vi "Ref_monitordata_struct_Add.vi"(6 "Active Sensors":bool[](array[boolean]), 8 "错误输入（无错误）":errorcluster, 9 "Controls[]":refnum<vi>[](array[refnum]), 10 "Ref_monitordata_struct":refnum<k24>[](array[refnum])) -> (0 "错误输出":errorcluster, 1 "Ref_monitordata_struct":refnum<k24>[](array[refnum]))   [LabVIEW 2017]
doc: "for reference monitor data"
uses:
  D:/test/PDLSTS/LV_PDL_Sample/DLL/STSProcess.dll
  DLL/STSProcess.dll
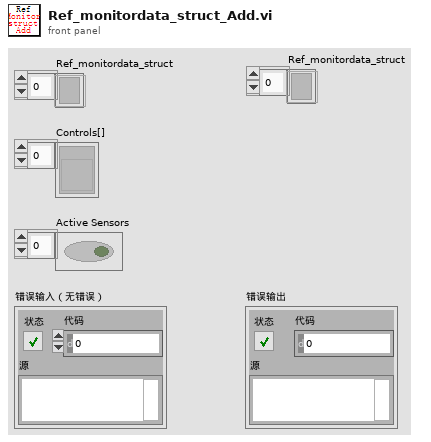
[diagram p1: front panel]
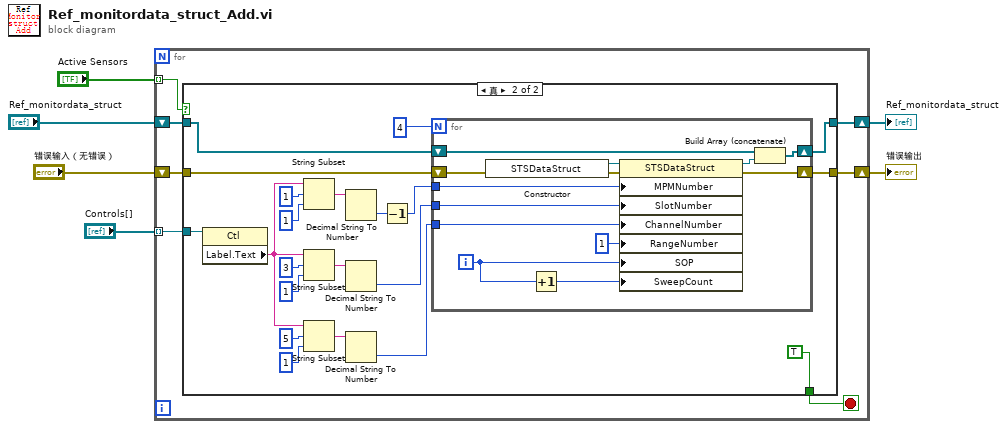
[diagram p0: block diagram]
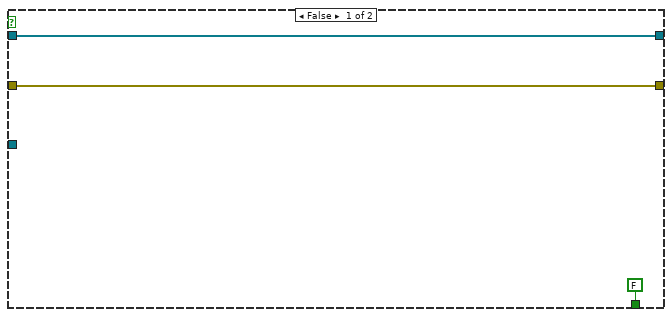
[diagram p2: hidden frame]
diagram:
  n1 = for {
    tunnel: "Controls[]" -> [w12] mode=indexing
    tunnel: "Active Sensors" -> [w13] mode=indexing
    shift-right: [w10] -> w4
    shift-left: "Ref_monitordata_struct" -> [w11]
    shift-right: [w8] -> w6
    shift-left: "错误输入（无错误）" -> [w9]
    stop <- w7 stop-if-true
    n2 = case shown="真" w13 {
      tunnel: w12 -> [_ w27]
      tunnel: w11 -> [w16 w18]
      tunnel: [w16 w22] -> w10
      tunnel: w9 -> [w15 w21]
      tunnel: [w15 w20] -> w8
      tunnel: [FALSE TRUE] -> w7
      frame False {
      }
      frame True {
        n3 = property class="Ctl"(reference=w27) -> ("Label.Text"=w26:string)  [unwired: 1 in, 2 out]
        n4 = String Subset(string=w26, offset (0)=1 ("偏移量(0)"), length (rest)=1 ("长度（剩余）")) -> (substring=w30:string)
        n5 = String Subset(string=w26, offset (0)=3 ("偏移量(0)"), length (rest)=1 ("长度（剩余）")) -> (substring=w31:string)
        n6 = String Subset(string=w26, offset (0)=5 ("偏移量(0)"), length (rest)=1 ("长度（剩余）")) -> (substring=w29:string)
        n7 = Decimal String To Number(string=w30) -> (number=w28:i32)  [unwired: 2 in, 1 out]
        n8 = Decimal String To Number(string=w31) -> (number=w24:i32)  [unwired: 2 in, 1 out]
        n9 = Decimal String To Number(string=w29) -> (number=w25:i32)  [unwired: 2 in, 1 out]
        n10 = Decrement(x=w28) -> (x-1=w23:i32)
        n11 = for {
          N: 4 -> [_]
          tunnel: w25 -> [w49]
          tunnel: w24 -> [w48]
          tunnel: w23 -> [w47]
          shift-right: [w50] -> w20
          shift-left: w21 -> [w44]
          shift-right: [w45] -> w22
          shift-left: w18 -> [w38]
          i -> [w43]
          n12 = constructor class="STSDataStruct"(error in=w44) -> (reference out=w41:refnum<k24>, error out=w42:errorcluster)  [unwired: 2 in, 1 out]
          n13 = Increment(x=w43) -> (x+1=w39:i32)
          n14 = property class="STSDataStruct"(reference=w41, error in=w42, "MPMNumber"=w47, "SlotNumber"=w48, "ChannelNumber"=w49, "RangeNumber"=1, "SOP"=w43, "SweepCount"=w39) -> (reference out=w46:refnum<k24>, error out=w50:errorcluster)
          n15 = Build Array (concatenate)(w38, w46) -> (w45:refnum<k24>[])
        }
      }
    }
  }
  "错误输出" <- w6
  "Ref_monitordata_struct" <- w4
